vi "Configure Targets Settings Dialog.vi"(11 "Targets Settings":T1) -> (2 "Cancelled":bool, 3 "Targets Settings":T1)   [LabVIEW 2020]
uses:
  Controls/Targets Settings.ctl
  Controls/FP Control Functions.ctl
  New folder/Globals.vi
panel:
  in  "Global Timeout (ms)":u32=4000
  in  "Reduce Discovery\nTimeout":bool
  in  "Cancel":bool
  in  "OK":bool
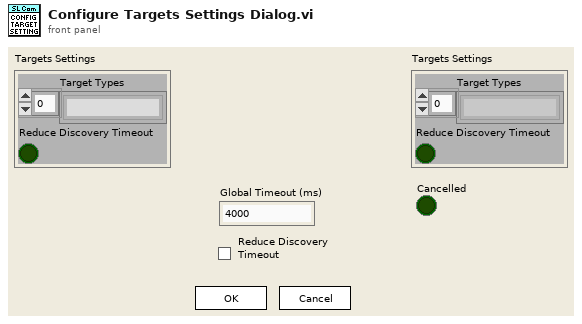
[diagram p1: front panel]
types:
  T1 = typedef "Targets Settings.ctl" = cluster{"Target Types":string[], "Reduce Discovery Timeout":bool}
  T2 = typedef "FP Control Functions.ctl" = enum16{"Open", "Close", "Bring To Front", "Center"}
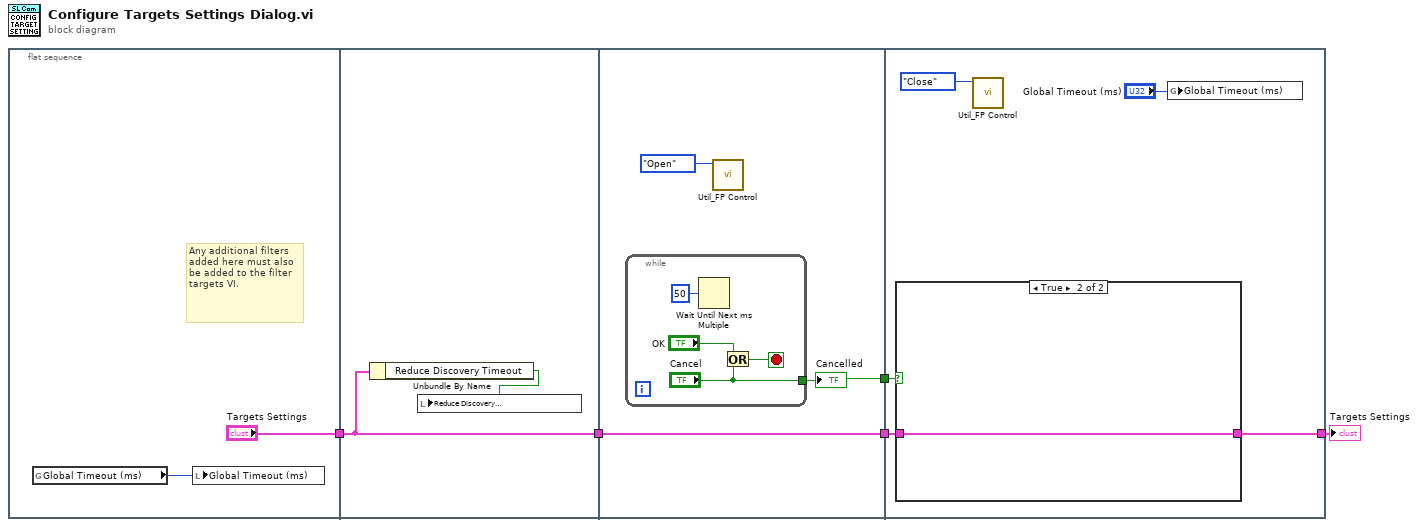
[diagram p0: block diagram]
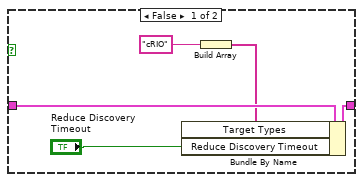
[diagram p2: hidden frame]
diagram:
  n1 = flat-sequence {
    tunnel: ["Targets Settings"] -> w1
    tunnel: [w9] -> w2
    tunnel: w1 -> [w9]
    tunnel: [w12] -> w5
    tunnel: [w11] -> w4
    tunnel: w2 -> [w11]
    tunnel: w5 -> [w21]
    tunnel: w4 -> [w20]
    tunnel: [w19] -> w3
    frame #0 {
      # "Any additional filters added here must also be added to the filter targets VI."
      n2 = global read "Globals.vi" "Global Timeout (ms)"() -> (w6:u32)
      n3 = local write "Global Timeout (ms)"(w6) -> ()
    }
    frame #1 {
      n4 = Unbundle By Name(w9) -> ("Reduce Discovery Timeout"=w8:bool)
      n5 = local write "Reduce Discovery\nTimeout"(w8) -> ()
    }
    frame #2 {
      n6 = while {
        tunnel: ["Cancel"] -> w12
        stop <- w14 stop-if-true
        n7 = Wait Until Next ms Multiple(millisecond multiple=u32 50) -> ()  [unwired: 1 out]
        n8 = Or(x="OK", y="Cancel") -> (x .or. y?=w14:bool)
      }
      "Cancelled" <- w12
      n9 = call "Util_FP Control.vi"("Function"=FP_Control_Functions."Open") -> ()  [unwired: 1 in, 10 out]
    }
    frame #3 {
      n10 = case shown="True" w21 {
        tunnel: w20 -> [w26 w27]
        tunnel: [w25 w27] -> w19
        frame False {
          n11 = Build Array("cRIO") -> (w22:string[])
          n12 = Bundle By Name(cluster=w26, "Target Types"=w22, "Reduce Discovery Timeout"="Reduce Discovery\nTimeout") -> (w25:T1)
        }
        frame True {
        }
      }
      n13 = call "Util_FP Control.vi"("Function"=FP_Control_Functions."Close") -> ()  [unwired: 1 in, 10 out]
      n14 = global write "Globals.vi" "Global Timeout (ms)"("Global Timeout (ms)") -> ()
    }
  }
  "Targets Settings" <- w3
